vi "Debug Board Viewer.vi"(0 "1D Board":T3[](array[typedef])=[{"Team"=0, "Occu."=enum."N", "Count"=0}, {"Team"=0, "Occu."=enum."N", "Count"=0}, {"Team"=1, "Occu."=enum."C", "Count"=1}, {"Team"=0, "Occu."=enum."N", "Count"=0}, {"Team"=1, "Occu."=enum."N", "Count"=1}, {"Team"=1, "Occu."=enum."C", "Count"=0}, {"Team"=1, "Occu."=enum."N", "Count"=1}, {"Team"=0, "Occu."=enum."N", "Count"=0}, {"Team"=0, "Occu."=enum."N", "Count"=0}, {"Team"=0, "Occu."=enum."N", "Count"=0}, {"Team"=0, "Occu."=enum."N", "Count"=0}, {"Team"=1, "Occu."=enum."K", "Count"=0}, {"Team"=1, "Occu."=enum."C", "Count"=2}, {"Team"=1, "Occu."=enum."C", "Count"=1}, {"Team"=0, "Occu."=enum."N", "Count"=0}, {"Team"=2, "Occu."=enum."C", "Count"=1}, {"Team"=0, "Occu."=enum."N", "Count"=0}, {"Team"=0, "Occu."=enum."N", "Count"=0}, {"Team"=0, "Occu."=enum."N", "Count"=0}, {"Team"=1, "Occu."=enum."C", "Count"=1}, {"Team"=0, "Occu."=enum."N", "Count"=0}, {"Team"=2, "Occu."=enum."C", "Count"=1}, {"Team"=2, "Occu."=enum."C", "Count"=1}, {"Team"=2, "Occu."=enum."C", "Count"=1}, {"Team"=2, "Occu."=enum."C", "Count"=1}, {"Team"=0, "Occu."=enum."N", "Count"=0}, {"Team"=0, "Occu."=enum."N", "Count"=0}, {"Team"=0, "Occu."=enum."N", "Count"=0}, {"Team"=2, "Occu."=enum."C", "Count"=1}, {"Team"=0, "Occu."=enum."N", "Count"=0}, {"Team"=1, "Occu."=enum."C", "Count"=1}, {"Team"=0, "Occu."=enum."N", "Count"=0}, {"Team"=1, "Occu."=enum."C", "Count"=1}, {"Team"=0, "Occu."=enum."N", "Count"=0}, {"Team"=0, "Occu."=enum."N", "Count"=0}, {"Team"=2, "Occu."=enum."C", "Count"=1}, {"Team"=0, "Occu."=enum."N", "Count"=0}, {"Team"=0, "Occu."=enum."N", "Count"=0}, {"Team"=0, "Occu."=enum."N", "Count"=0}, {"Team"=0, "Occu."=enum."N", "Count"=0}, {"Team"=0, "Occu."=enum."N", "Count"=0}, {"Team"=1, "Occu."=enum."C", "Count"=1}, {"Team"=0, "Occu."=enum."N", "Count"=0}, {"Team"=0, "Occu."=enum."N", "Count"=0}, {"Team"=1, "Occu."=enum."C", "Count"=1}, {"Team"=1, "Occu."=enum."C", "Count"=1}, {"Team"=0, "Occu."=enum."N", "Count"=0}, {"Team"=0, "Occu."=enum."N", "Count"=0}, {"Team"=0, "Occu."=enum."N", "Count"=0}], 5 "Show Cell Index?":bool) -> (4 "Debug Board":T2, 6 "Debug Board 2D String":T1)   [LabVIEW 2014]
uses:
  Typedefs/Board Cell.ctl
  Typedefs/Cell Occupancy.ctl
  Typedefs/Debug Board View.ctl
  Typedefs/Debug Board 2D String.ctl
  Dragon Tamers.lvlib
panel:
  out "Array":dbl[](array[numeric])
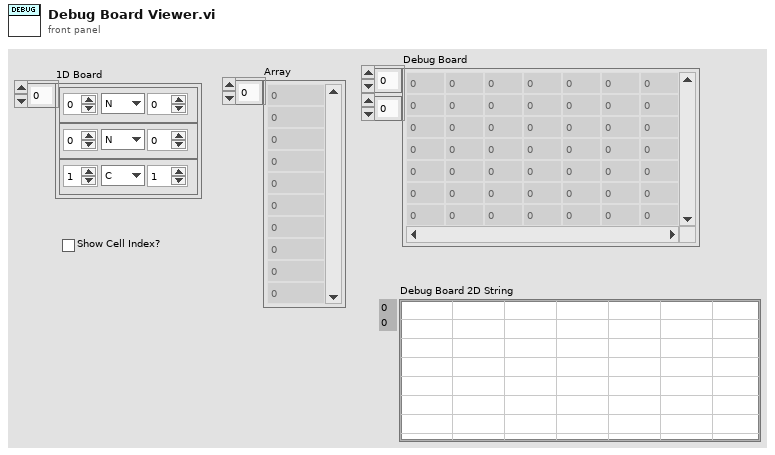
[diagram p1: front panel]
types:
  T1 = typedef "Dragon Tamers.lvlib/Debug Board 2D String.ctl" = string[][]
  T2 = typedef "Debug Board View.ctl" = dbl[][]
  T3 = typedef "Dragon Tamers.lvlib/Board Cell.ctl" = cluster{"Team":i32, "Occu.":T4, "Count":i32}
  T4 = typedef "Dragon Tamers.lvlib/Cell Occupancy.ctl" = enum16{"N", "C", "K"}
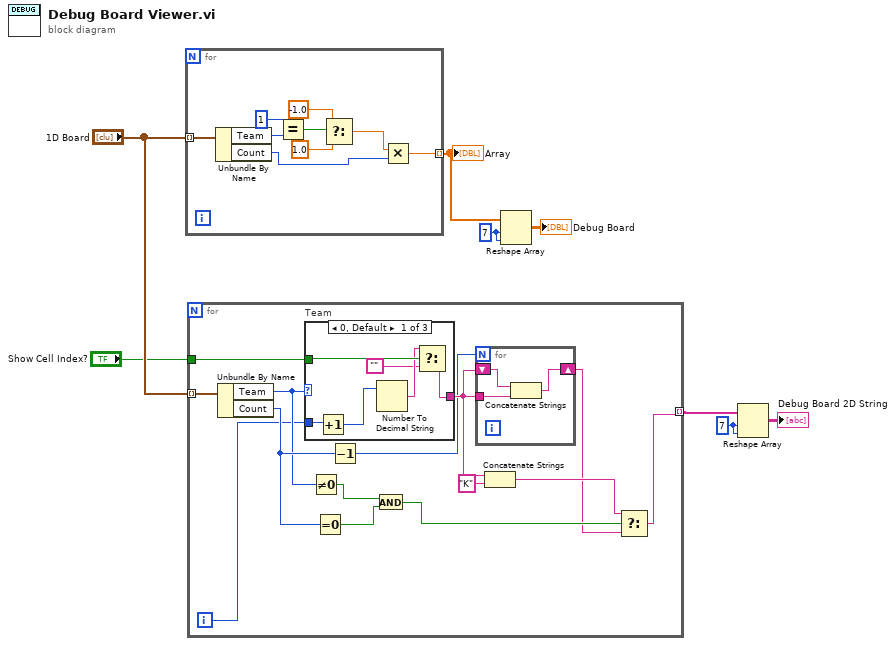
[diagram p0: block diagram]
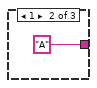
[diagram p2: hidden frame]
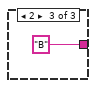
[diagram p3: hidden frame]
diagram:
  w4 = 7 ("dimension size")
  w8 = 7 ("dimension size")
  n1 = for {
    tunnel: "1D Board" -> [w17] mode=indexing
    tunnel: [w9] -> w7 mode=indexing
    n2 = Unbundle By Name(w17) -> ("Team"=w16:i32, "Count"=w10:i32)
    n3 = Equal?(x=1, y=w16) -> (x = y?=w14:bool)
    n4 = Select(t=-1.0, s=w14, f=1.0) -> (s? t:f=w11:dbl)
    n5 = Multiply(x=w11, y=w10) -> (x*y=w9:dbl)
  }
  "Array" <- w7
  n6 = for {
    tunnel: "1D Board" -> [w31] mode=indexing
    tunnel: [w22] -> w3 mode=indexing
    tunnel: "Show Cell Index?" -> [w18]
    i -> [w19]
    n7 = Unbundle By Name(w31) -> ("Team"=w26:i32, "Count"=w28:i32)
    n8 = case "Team" shown="0, Default" w26 {
      tunnel: [w36 "A" "B"] -> w21
      tunnel: w19 -> [w40 _ _]
      tunnel: w18 -> [w38 _ _]
      frame 0, Default {
        n9 = Increment(x=w40) -> (x+1=w39:i32)
        n10 = Number To Decimal String(number=w39) -> (decimal integer string=w37:string)  [unwired: 1 in]
        n11 = Select(t=w37, s=w38, f="") -> (s? t:f=w36:string)
      }
      frame 1 {
      }
      frame 2 {
      }
    }
    n12 = Not Equal To 0?(x=w26) -> (x != 0?=w30:bool)
    n13 = Equal To 0?(x=w28) -> (x = 0?=w29:bool)
    n14 = Decrement(x=w28) -> (x-1=w20:i32)
    n15 = And(x=w30, y=w29) -> (x .and. y?=w27:bool)
    n16 = for {
      N: w20 -> [_]
      tunnel: w21 -> [w34]
      shift-right: [w33] -> w23
      shift-left: w21 -> [w32]
      n17 = Concatenate Strings(w32, w34) -> (w33:string)
    }
    n18 = Concatenate Strings(w21, "K" ("string")) -> (w24:string)
    n19 = Select(t=w24, s=w27, f=w23) -> (s? t:f=w22:string)
  }
  n20 = Reshape Array(w7, w8, w8) -> (→"Debug Board":dbl[][])
  n21 = Reshape Array(w3, w4, w4) -> (→"Debug Board 2D String":string[][])
